vi "RX.vi"() -> ()   [LabVIEW 2020]
panel:
  in  "RX":dbl
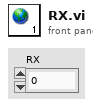
[diagram p1: front panel]
diagram:
